vi "Playback Controls.vi"() -> ()   [LabVIEW 2017]
uses:
  <vilib>/Rock Robotics/WPI/Dashboard/WPI_DashboardPlay Operation.ctl
  <vilib>/Rock Robotics/WPI/Dashboard/WPI_DashboardLogging Global.vi
  <vilib>/Utility/inputDevices.llb/mouseAcquire.vi
panel:
  in  "Operation":u16(ring) items=["", "Rename", "Delete", "Show Folder"]
  in  "Rename":string
  in  "Dragging?":bool
  in  "Scrollbar":dbl(slide) scale=0.0..12.36
  in  "Speed":u16(ring)=3 items=["1/10 x", "1/5 x", "1/2 x", "1 x", "2 x", "5 x", "10 x"]
  in  "Playback Button":bool
  in  "Pause Button":bool
  in  "File Selector":u16(ring) items=["Select a Log File", "2017_11_07 07-17-37 Tue -- 3.2 secs", "2017_11_07 08-09-29 Tue -- 8.7 secs", "2017_11_07 08-19-10 Tue -- 11.1 secs", "2017_11_07 08-21-00 Tue -- 12.4 secs", "Test -- 2.6 secs"]
  in  "Drag Button":bool
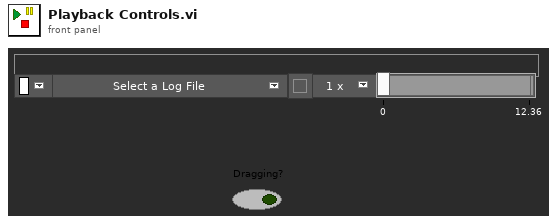
[diagram p1: front panel]
types:
  T1 = typedef "WPI_DashboardPlay Operation.ctl" = enum16{"Play", "Pause", "Finished"}
  T2 = typedef "LVRectTypeDef.ctl" = cluster{"Left":i16, "Top":i16, "Right":i16, "Bottom":i16}
  T3 = cluster{"Horizontal":i32, "Vertical":i32, "Scrolling":i32}
  T4 = cluster{"Horizontal":i32, "Vertical":i32, "Horizontal":i32, "Vertical":i32}
  T5 = cluster{"button 1":bool, "button 2":bool, "button 3":bool, "button 4":bool}
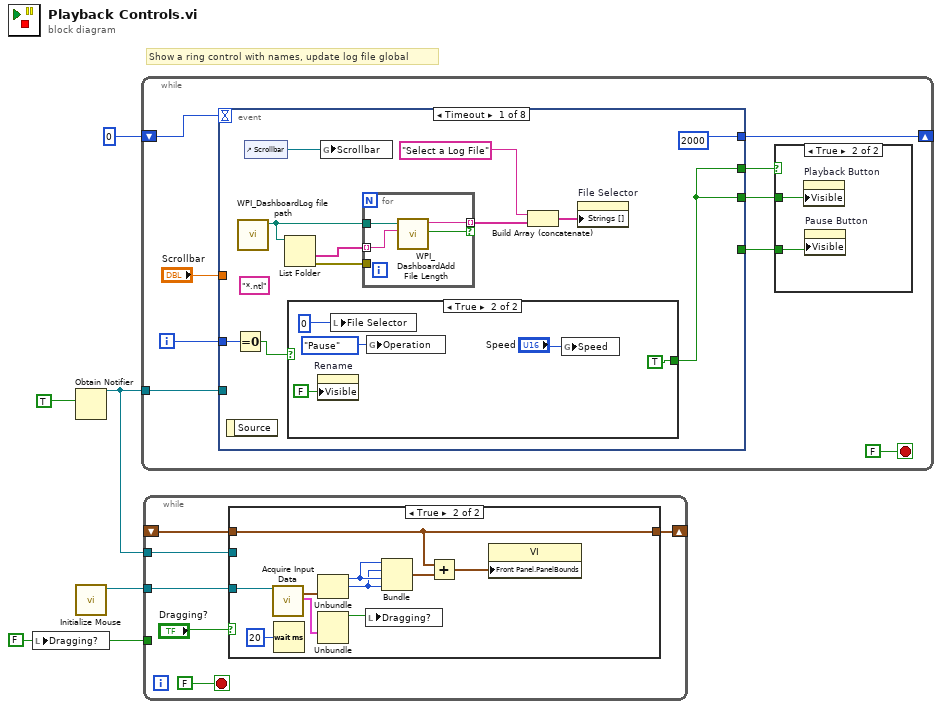
[diagram p0: block diagram]
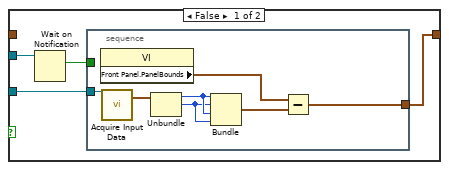
[diagram p2: hidden frame]
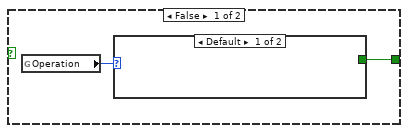
[diagram p4: hidden frame]
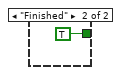
[diagram p5: hidden frame]
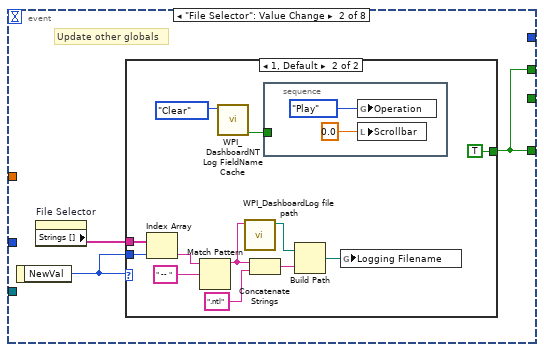
[diagram p6: hidden frame]
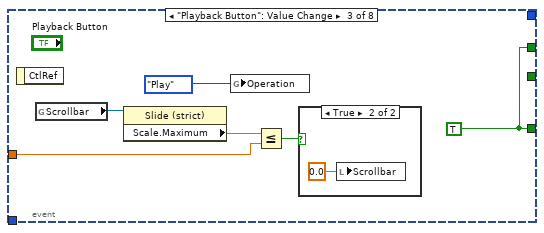
[diagram p8: hidden frame]
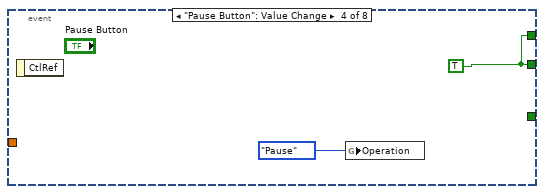
[diagram p10: hidden frame]
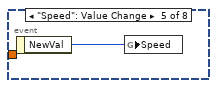
[diagram p11: hidden frame]
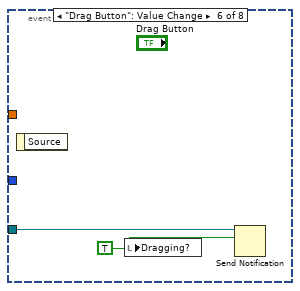
[diagram p12: hidden frame]
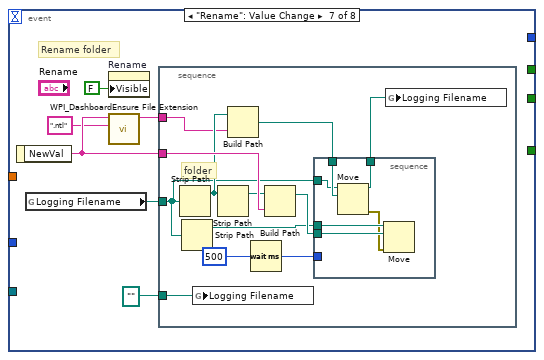
[diagram p13: hidden frame]
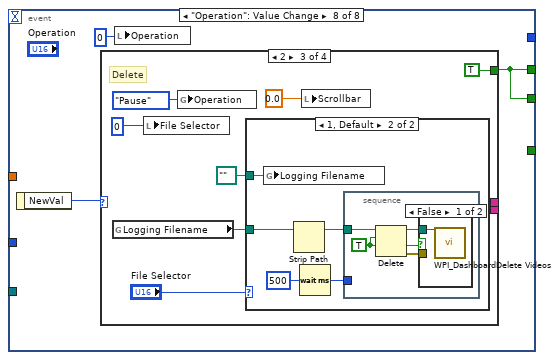
[diagram p14: hidden frame]
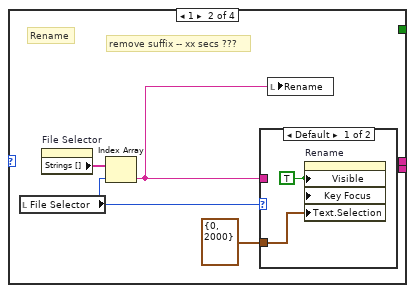
[diagram p16: hidden frame]
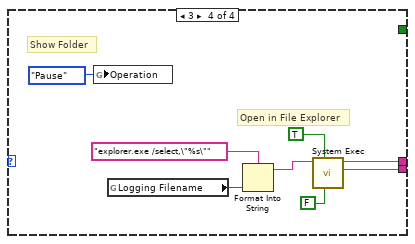
[diagram p20: hidden frame]
diagram:
  w2 = FALSE ("Dragging?")
  # "Show a ring control with names, update log file global"
  n1 = local write "Dragging?"(w2) -> ()
  n2 = Obtain Notifier(notification data type=TRUE ("Dragging?")) -> (notifier out=w3:refnum<notifier>)  [unwired: 3 in, 2 out]
  n3 = call <vilib>:"Initialize Mouse.vi"() -> ("device ID"=w4:refnum<k1>)  [unwired: 10 in, 1 out]
  n4 = while {
    shift-right: [w13] -> _
    shift-left: 0 -> [w12]
    tunnel: w3 -> [w6]
    i -> [w8]
    stop <- FALSE stop-if-true
    n5 = event shown="[0] Timeout" {
      selector: _ -> [_ _ _ _ _ _ _ _]
      dyn-events: _ -> [_ _ _ _ _ _ _ _]
      timeout: w12 -> [_ _ _ _ _ _ _ _]
      tunnel: [2000 _ _ _ _ _ _ _] -> w13
      tunnel: [_ w40 w62 _ _ _ _ _] -> w11
      tunnel: [w20 _ _ w65 _ _ _ w94] -> w10
      tunnel: [w20 w40 w62 w65 _ _ _ w94] -> w9
      tunnel: w8 -> [w22 _ _ _ _ _ _ _]
      tunnel: "Scrollbar" -> [_ _ w58 _ _ _ _ _]
      tunnel: w6 -> [_ _ _ _ _ w68 _ _]
      event Timeout {
        (unwired) "*.ntl" ("pattern")
        n6 = event-data() -> ()  [unwired: 1 in, 1 out]
        n7 = Equal To 0?(x=w22) -> (x = 0?=w21:bool)
        n8 = call <vilib>:"WPI_DashboardLog file path.vi"() -> ("appended path"=w19:path)  [unwired: 11 in]
        n9 = control-ref of="Scrollbar"() -> (w26:refnum<vi>)
        n10 = List Folder(path=w19) -> (folder names=w17:string[], error out=w18:errorcluster)  [unwired: 3 in, 2 out]
        n11 = case shown="True" w21 {
          tunnel: [w28 TRUE] -> w20
          frame False {
            n12 = global read "WPI_DashboardLogging Global.vi" "Operation"() -> (w29:T1)
            n13 = case shown="Default" w29 {
              tunnel: [_ TRUE] -> w28
              frame Default {
              }
              frame "Finished" {
              }
            }
          }
          frame True {
            n14 = property on="Rename" class="Str"("Visible"=FALSE) -> ()  [unwired: 2 in, 2 out]
            n15 = local write "File Selector"(0) -> ()
            n16 = global write "WPI_DashboardLogging Global.vi" "Operation"(WPI_DashboardPlay_Operation."Pause" ("Operation")) -> ()
            n17 = global write "WPI_DashboardLogging Global.vi" "Speed"("Speed") -> ()
          }
        }
        n18 = global write "WPI_DashboardLogging Global.vi" "Scrollbar"(w26) -> ()
        n19 = for {
          tunnel: w17 -> [w37] mode=indexing
          tunnel: [w39] -> w25 mode=indexing if=w36
          tunnel: w19 -> [w38]
          tunnel: w18 -> [_]
          n20 = call <vilib>:"WPI_DashboardAdd File Length.vi"("String in"=w37, "appended path"=w38) -> ("Valid"=w36:bool, "String out"=w39:string)  [unwired: 8 in]
        }
        n21 = Build Array (concatenate)("Select a Log File" ("pattern"), w25) -> (w24:string[])
        n22 = property on="File Selector" class="Ring (strict)"("Strings []"=w24) -> ()  [unwired: 2 in, 2 out]
      }
      event "File Selector": Value Change {
        # "Update other globals"
        n23 = event-data() -> ("NewVal"=w41:u16)  [unwired: 1 in]
        n24 = property on="File Selector" class="Ring (strict)"() -> ("Strings []"=w42:string[])  [unwired: 2 in, 2 out]
        n25 = case shown="1, Default" w41 {
          tunnel: w42 -> [_ w54]
          tunnel: w41 -> [_ w53]
          tunnel: [_ TRUE ("Visible")] -> w40
          frame 0 {
          }
          frame 1, Default {
            n26 = Index Array(array=w54, index=w53) -> (element=w48:string)
            n27 = Match Pattern(string=w48, regular expression=" -- ") -> (before substring=w43:string)  [unwired: 1 in, 3 out]
            n28 = call <vilib>:"WPI_DashboardNT Log FieldName Cache.vi"("Operation"=enum16{"Lookup/Add", "Index", "Clear"}."Clear") -> ("New/Valid"=w45:bool)  [unwired: 8 in, 2 out]
            n29 = call <vilib>:"WPI_DashboardLog file path.vi"("Time Date String"=w43) -> ("appended path"=w52:path)  [unwired: 10 in]
            n30 = Concatenate Strings(w43, ".ntl") -> (w50:string)
            n31 = stacked-sequence {
              tunnel: w45 -> [_]
              frame #0 {
                n32 = global write "WPI_DashboardLogging Global.vi" "Operation"(WPI_DashboardPlay_Operation."Play" ("Operation")) -> ()
                n33 = local write "Scrollbar"(0.0 ("Position")) -> ()
              }
            }
            n34 = Build Path(base path=w52, name or relative path=w50) -> (appended path=w49:path)
            n35 = global write "WPI_DashboardLogging Global.vi" "Logging Filename"(w49) -> ()
          }
        }
      }
      event "Playback Button": Value Change {
        w62 = TRUE ("Visible")
        n36 = event-data() -> ()  [unwired: 1 in, 1 out]
        n37 = global read "WPI_DashboardLogging Global.vi" "Scrollbar"() -> (w60:refnum<vi>)
        n38 = property class="Slide (strict)"(reference=w60) -> ("Scale.Maximum"=w59:dbl)  [unwired: 1 in, 2 out]
        n39 = global write "WPI_DashboardLogging Global.vi" "Operation"(WPI_DashboardPlay_Operation."Play" ("Operation")) -> ()
        n40 = Less Or Equal?(x=w59, y=w58) -> (x <= y?=w57:bool)
        n41 = case shown="True" w57 {
          frame False {
          }
          frame True {
            n42 = local write "Scrollbar"(0.0 ("Scrollbar")) -> ()
          }
        }
      }
      event "Pause Button": Value Change {
        w65 = TRUE ("Visible")
        n43 = event-data() -> ()  [unwired: 1 in, 1 out]
        n44 = global write "WPI_DashboardLogging Global.vi" "Operation"(WPI_DashboardPlay_Operation."Pause" ("Operation")) -> ()
      }
      event "Speed": Value Change {
        n45 = event-data() -> ("NewVal"=w66:u16)  [unwired: 1 in]
        n46 = global write "WPI_DashboardLogging Global.vi" "Speed"(w66) -> ()
      }
      event "Drag Button": Value Change {
        w67 = TRUE ("Dragging?")
        n47 = event-data() -> ()  [unwired: 1 in, 1 out]
        n48 = local write "Dragging?"(w67) -> ()
        n49 = Send Notification(notification=w67, notifier=w68) -> ()  [unwired: 1 in, 2 out]
      }
      event "Rename": Value Change {
        # "Rename folder"
        n50 = event-data() -> ("NewVal"=w71:string)  [unwired: 1 in]
        n51 = global read "WPI_DashboardLogging Global.vi" "Logging Filename"() -> (w73:path)
        n52 = property on="Rename" class="Str"("Visible"=FALSE) -> ()  [unwired: 2 in, 2 out]
        n53 = call <vilib>:"WPI_DashboardEnsure File Extension.vi"("Extension"=".ntl", "Name"=w71) -> ("Name Out"=w69:string)  [unwired: 9 in]
        n54 = stacked-sequence {
          tunnel: w71 -> [w82]
          tunnel: w73 -> [w75]
          tunnel: path "" ("Logging Filename") -> [w85]
          tunnel: w69 -> [w77]
          frame #0 {
            # "folder"
            n55 = Strip Path(path=w75) -> (stripped path=w78:path)  [unwired: 1 out]
            n56 = Strip Path(path=w75) -> (stripped path=w79:path)  [unwired: 1 out]
            n57 = global write "WPI_DashboardLogging Global.vi" "Logging Filename"(w85) -> ()
            n58 = Strip Path(path=w78) -> (stripped path=w80:path)  [unwired: 1 out]
            n59 = Build Path(base path=w78, name or relative path=w77) -> (appended path=w76:path)
            n60 = Wait (ms)(milliseconds to wait=u32 500) -> (millisecond timer value=w83:u32)
            n61 = Build Path(base path=w80, name or relative path=w82) -> (appended path=w86:path)
            n62 = stacked-sequence {
              tunnel: w86 -> [w92]
              tunnel: w79 -> [w91]
              tunnel: w83 -> [_]
              tunnel: [w89] -> w81
              tunnel: w76 -> [w90]
              tunnel: w75 -> [w88]
              frame #0 {
                n63 = Move(source path=w88, 10:w90) -> (error out=w87:errorcluster, 3:w89:path)  [unwired: 3 in, 1 out]
                n64 = Move(source path=w91, error in=w87, 10:w92) -> ()  [unwired: 2 in, 3 out]
              }
            }
            n65 = global write "WPI_DashboardLogging Global.vi" "Logging Filename"(w81) -> ()
          }
        }
      }
      event "Operation": Value Change {
        n66 = event-data() -> ("NewVal"=w95:u16)  [unwired: 1 in]
        n67 = case shown="2" w95 {
          tunnel: [_ _ TRUE _] -> w94
          tunnel: [_ _ _ w123] -> _
          tunnel: [_ _ _ w122] -> _
          frame 0, Default {
          }
          frame 1 {
            # "remove suffix -- xx secs ???"
            # "Rename"
            n68 = local read "File Selector"() -> (w97:u16)
            n69 = property on="File Selector" class="Ring (strict)"() -> ("Strings []"=w99:string[])  [unwired: 2 in, 2 out]
            n70 = Index Array(array=w99, index=w97) -> (element=w98:string)
            n71 = case shown="Default" w97 {
              tunnel: w98 -> [_ _]
              tunnel: cluster{i32, i32} {0, 2000} -> [w100 _]
              frame Default {
                w101 = TRUE ("Visible")
                n72 = property on="Rename" class="Str"("Visible"=w101, "Key Focus"=w101, "Text.Selection"=w100) -> ()  [unwired: 2 in, 2 out]
              }
              frame 0 {
              }
            }
            n73 = local write "Rename"(w98) -> ()
          }
          frame 2 {
            # "Delete"
            n74 = global read "WPI_DashboardLogging Global.vi" "Logging Filename"() -> (w104:path)
            n75 = local write "File Selector"(0) -> ()
            n76 = global write "WPI_DashboardLogging Global.vi" "Operation"(WPI_DashboardPlay_Operation."Pause" ("Operation")) -> ()
            n77 = case shown="1, Default" "File Selector" {
              tunnel: w104 -> [_ w110]
              tunnel: path "" ("Logging Filename") -> [_ w113]
              frame 0 {
              }
              frame 1, Default {
                n78 = global write "WPI_DashboardLogging Global.vi" "Logging Filename"(w113) -> ()
                n79 = Strip Path(path=w110) -> (stripped path=w109:path)  [unwired: 1 out]
                n80 = Wait (ms)(milliseconds to wait=u32 500) -> (millisecond timer value=w111:u32)
                n81 = stacked-sequence {
                  tunnel: w109 -> [w118]
                  tunnel: w111 -> [_]
                  frame #0 {
                    w115 = TRUE ("confirm (F)")
                    n82 = Delete(path (use dialog)=w118, entire hierarchy (F)=w115, confirm (F)=w115) -> (deleted path=w116:path, cancelled=w117:bool, error out=w114:errorcluster)  [unwired: 2 in]
                    n83 = case shown="False" w117 {
                      tunnel: w116 -> [w119 _]
                      tunnel: w114 -> [_ _]
                      frame False {
                        n84 = call <vilib>:"WPI_DashboardDelete Videos.vi"("Path"=w119) -> ()  [unwired: 11 in]
                      }
                      frame True {
                      }
                    }
                  }
                }
              }
            }
            n85 = local write "Scrollbar"(0.0 ("Position")) -> ()
          }
          frame 3 {
            # "Open in File Explorer"
            # "Show Folder"
            n86 = global write "WPI_DashboardLogging Global.vi" "Operation"(WPI_DashboardPlay_Operation."Pause" ("Operation")) -> ()
            n87 = global read "WPI_DashboardLogging Global.vi" "Logging Filename"() -> (w120:path)
            n88 = Format Into String(format string="explorer.exe /select,\"%s\"", w120) -> (resulting string=w126:string)  [unwired: 2 in, 1 out]
            n89 = call <vilib>:"System Exec.vi"("run minimized? (F)"=FALSE, "wait until completion? (T)"=TRUE, "command line"=w126) -> ("standard error"=w123:string, "standard output"=w122:string)  [unwired: 5 in, 2 out]
          }
        }
        n90 = local write "Operation"(0) -> ()
      }
    }
    n91 = case shown="True" w9 {
      tunnel: w11 -> [_ w16]
      tunnel: w10 -> [_ w15]
      frame False {
      }
      frame True {
        n92 = property on="Playback Button" class="Bool"("Visible"=w15) -> ()  [unwired: 2 in, 2 out]
        n93 = property on="Pause Button" class="Bool"("Visible"=w16) -> ()  [unwired: 2 in, 2 out]
      }
    }
  }
  n94 = while {
    tunnel: w4 -> [w133]
    tunnel: w3 -> [w131]
    tunnel: w2 -> [_]
    shift-right: [w129] -> _
    shift-left: _ -> [w128]
    stop <- FALSE stop-if-true
    n95 = case shown="True" "Dragging?" {
      tunnel: w133 -> [w136 w154]
      tunnel: w131 -> [w137 _]
      tunnel: [w135 w146] -> w129
      tunnel: w128 -> [_ w146]
      frame False {
        n96 = Wait on Notification(notifier=w137) -> (notification=w134:bool)  [unwired: 3 in, 3 out]
        n97 = stacked-sequence {
          tunnel: w136 -> [w144]
          tunnel: [w140] -> w135
          tunnel: w134 -> [_]
          frame #0 {
            n98 = property class="VI"() -> ("Front Panel.PanelBounds"=w142:T2)  [unwired: 2 in, 2 out]
            n99 = call-poly <vilib>:"Acquire Input Data.vi"("device ID"=w144) -> ("axis info"=w143:T3)  [unwired: 15 in, 3 out]
            n100 = Unbundle(w143) -> ("Horizontal"=w139:i32, "Vertical"=w138:i32)  [unwired: 1 out]
            n101 = Bundle("Horizontal"=w139, "Vertical"=w138, "Horizontal"=w139, "Vertical"=w138) -> (w141:T4)  [unwired: 1 in]
            n102 = Subtract(x=w142, y=w141) -> (x-y=w140:cluster{i32, i32, i32, i32})
          }
        }
      }
      frame True {
        n103 = call-poly <vilib>:"Acquire Input Data.vi"("device ID"=w154) -> ("axis info"=w150:T3, "button info"=w152:T5)  [unwired: 15 in, 2 out]
        n104 = Wait (ms)(milliseconds to wait=u32 20) -> ()  [unwired: 1 out]
        n105 = Unbundle(w150) -> ("Horizontal"=w149:i32, "Vertical"=w148:i32)  [unwired: 1 out]
        n106 = Unbundle(w152) -> ("button 1"=w151:bool)  [unwired: 3 out]
        n107 = local write "Dragging?"(w151) -> ()
        n108 = Bundle("Horizontal"=w149, "Vertical"=w148, "Horizontal"=w149, "Vertical"=w148) -> (w147:T4)  [unwired: 1 in]
        n109 = Add(x=w146, y=w147) -> (x+y=w145:cluster{i32, i32, i32, i32})
        n110 = property class="VI"("Front Panel.PanelBounds"=w145) -> ()  [unwired: 2 in, 2 out]
      }
    }
  }
